vi "GraphSetting Conv MapMode.vi"(11 "ログ":bool) -> (3 "Xスケール.マッピングモード":u8)   [LabVIEW 2014]
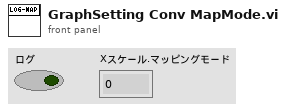
[diagram p1: front panel]
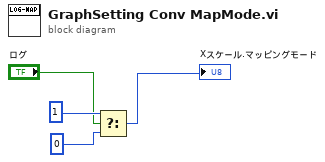
[diagram p0: block diagram]
diagram:
  n1 = Select(t=u8 1 ("Xスケール.マッピングモード"), s="ログ", f=u8 0 ("Xスケール.マッピングモード")) -> (s? t:f=→"Xスケール.マッピングモード":u8)
